vi "Agilent PNA Series Catalog Measurements.vi"(0 "VISA Resource Name":refnum<visa-resource-name>, 5 "Channel (1)":i32=1, 7 "Display Window (1)":i32=1) -> (6 "Measurement Parameter Array":string[][](array[string]), 8 "Window Array":i32[](array[numeric]), 10 "Trace Array":i32[](array[numeric]))   [LabVIEW 2014]
doc: "This VI catalogs the currently defined measurements, windows, and traces, selects a measurement for further definition and adds a title to the window."
uses:
  Agilent PNA Series.lvlib
panel:
  # "(c) 2005-2015 National Instruments.  ALL RIGHTS RESERVED."
  # "Meas Name"
  # "Meas Type"
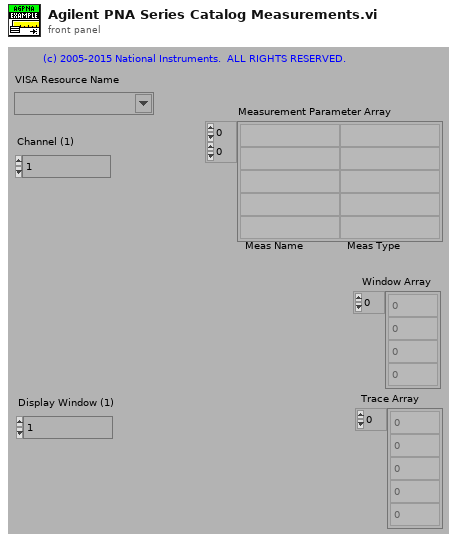
[diagram p1: front panel]
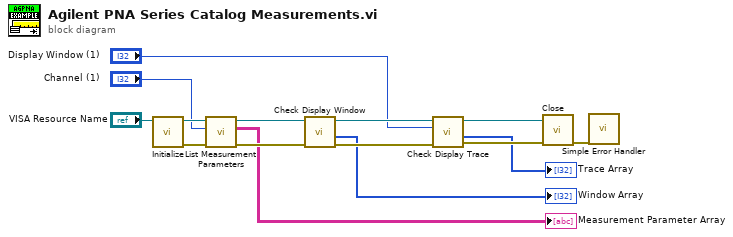
[diagram p0: block diagram]
diagram:
  n1 = call "Initialize.vi"("Instrument Resource Name"="VISA Resource Name") -> ("error out"=w2:errorcluster, "dup VISA session"=w15:refnum<visa-resource-name>)  [unwired: 9 in]
  n2 = call "List Measurement Parameters.vi"("Error In (no error)"=w2, "Channel (1)"="Channel (1)", "VISA Resource Name"=w15) -> ("Error Out"=w12:errorcluster, "Measurement Parameter Array"=→"Measurement Parameter Array":string[][], "VISA Resource Name Out"=w13:refnum<visa-resource-name>)  [unwired: 6 in]
  n3 = call "Check Display Window.vi"("Error In (no error)"=w12, "VISA Resource Name"=w13) -> ("Error Out"=w11:errorcluster, "Window Array"=→"Window Array":i32[], "VISA Resource Name Out"=w10:refnum<visa-resource-name>)  [unwired: 6 in, 1 out]
  n4 = call "Check Display Trace.vi"("Error In (no error)"=w11, "Display Window (1)"="Display Window (1)", "VISA Resource Name"=w10) -> ("Error Out"=w14:errorcluster, "Trace Array"=→"Trace Array":i32[], "VISA Resource Name Out"=w4:refnum<visa-resource-name>)  [unwired: 5 in, 1 out]
  n5 = call "Close.vi"("Error In (no error)"=w14, "VISA Resource Name"=w4) -> ("Error Out"=w3:errorcluster)  [unwired: 9 in]
  n6 = call <vilib>:"Simple Error Handler.vi"("error in (no error)"=w3) -> ()  [unwired: 4 in, 5 out]
